vi "Hololens_GaitDisplay.vi"() -> ()   [LabVIEW 2016]
doc: "VI demonstrating how to add 3D objects to the Hololens space and to 3D Picture controls.\n\nHaro3D 2.2.0.7\nCopyright (c) 2018, HaroTek"
uses:
  Program Files (x86)/National Instruments/LabVIEW 2016/examples/HaroTek/Haro3D Examples/controls/_Hololens_3dobject_example_tab.ctl
  <vilib>/Utility/miscctls.llb/LV3DPointTypeDef.ctl
  <vilib>/HaroTek/Haro3D/Utilities/3D objects/controls/Material_info.ctl
  Program Files (x86)/National Instruments/LabVIEW 2016/examples/HaroTek/Haro3D Examples/Support/Holo_Example_Shape_ref_typedef.ctl
  <vilib>/HaroTek/Haro3D/Utilities/3D objects/3D_Shape_class/3D_Shape.lvclass
  C:/Program Files (x86)/National Instruments/LabVIEW 2016/vi.lib/HaroTek/Haro3D/Utilities/3D objects/3D_Object_class/3D_Object.lvclass
  <vilib>/HaroTek/Haro3D/Utilities/3D Operations/controls/_Deg_Rad_typedef.ctl
  <vilib>/HaroTek/Haro3D/Utilities/3D objects/Box_class/3D_Box.lvclass
  C:/Program Files (x86)/National Instruments/LabVIEW 2016/vi.lib/HaroTek/Haro3D/Utilities/3D objects/3D_Shape_class/3D_Shape.lvclass
  <vilib>/HaroTek/Haro3D/Utilities/3D objects/Cylinder_class/3D_Cylinder.lvclass
  <vilib>/HaroTek/Haro3D/Utilities/3D objects/Sphere_class/3D_Sphere_class/3D_Sphere.lvclass
  <vilib>/HaroTek/Haro3D/Utilities/3D objects/Mesh_class/Mesh.lvclass
  <vilib>/HaroTek/Haro3D/Utilities/3D objects/3D_Quad_class/Panel.lvclass
  <vilib>/picture/3D Picture Control/Object/Create Object (name).vi
  <vilib>/HaroTek/Haro3D/Utilities/3D objects/3D_Shape_class/properties/WriteMaterialInfo.vi
  <vilib>/HaroTek/Haro3D/Utilities/3D objects/3D_Object_class/properties/WritePosition.vi
  <vilib>/picture/3D Picture Control/Object/Add Object (reference).vi
  <vilib>/HaroTek/Haro3D/Utilities/3D objects/3D_Object_class/properties/ReadOrientation.vi
  <vilib>/HaroTek/Haro3D/Utilities/3D objects/OBJ classes/OBJ_Mesh_class/properties/ReadMeshArray.vi
  <vilib>/HaroTek/Haro3D/Utilities/3D objects/3D_Shape_class/properties/ReadShape.vi
  <vilib>/HaroTek/Haro3D/Utilities/3D objects/3D_Object_class/properties/ReadPosition.vi
  <vilib>/HaroTek/Haro3D/Utilities/3D objects/OBJ classes/OBJ_Mesh_class/OBJ_Mesh.lvclass
  <vilib>/HaroTek/Haro3D/Haro3D.lvlib
  <vilib>/picture/3D Picture Control/NI_3D Picture Control.lvlib
  <vilib>/HaroTek/Haro3D/Hololens/Hololens_class/Hololens.lvclass
  <vilib>/HaroTek/Haro3D/Hololens/Modules/Hololens Message classes/Object_Selected_Message_class/Object_Selected_Message.lvclass
  <vilib>/HaroTek/Haro3D/Hololens/Modules/Hololens Message classes/Mesh_Message_class/Mesh_Message.lvclass
panel:
  in  "Control container":enum32{"Page 2"}(tab)
  in  "Color":u32(colorbox)=16711680
  in  "Tab Control":T1
  in  "Cyl Length":sgl=0.3
  in  "Add Cylinder":bool
  in  "Cyl Radius":sgl=0.1
  in  "Cylinder info":string="Cylinder created in \nLabVIEW!"
  in  "Add Box":bool
  in  "Dimensions":T2={"X"=0.3, "Y"=0.2, "Z"=0.1}
  in  "Box Info":string="Box created in \nLabVIEW!"
  in  "Sphere Diameter":sgl=0.4
  in  "Add Sphere":bool
  in  "Sphere info":string="Sphere created in \nLabVIEW!"
  in  "Add Mesh":bool
  in  "Scale":dbl=1.0 format="%#_13g"
  in  "Panel":bool
  in  "Position":T2={"X"=0.0, "Y"=0.0, "Z"=2.0}
  in  "X rotation":sgl(slide) scale=-90.0..90.0
  in  "Y rotation":sgl(slide) scale=-180.0..270.0
  in  "Z rotation":sgl(slide) scale=-90.0..90.0
  in  "Pointer":bool
  in  "Reset View":bool
  out "Hololens":bool
  out "3D Picture":refnum<vi>(3d-picture)
  # "1. Start this VI and the Haro3D app on the Hololens\n2. Wait until the Hololens is connected to this VI.\n3. Use the tab to select a 3D object.\n4. Click to add the object to the Hololens and 3D Pict control\n5. Click again to modify the object properties\n6. Click the X to terminate the VI and the Hololens app."
  # "www.harotek.com"
  # "Scale is applied only when adding the mesh."
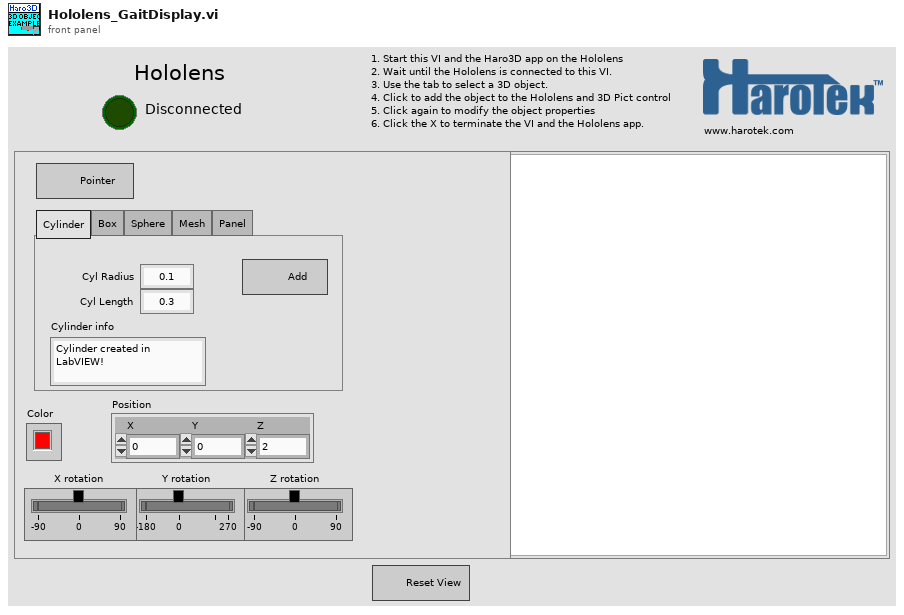
[diagram p1: front panel]
types:
  T1 = typedef "_Hololens_3dobject_example_tab.ctl" = enum32{"Cylinder", "Box", "Sphere", "Mesh", "Panel"}
  T2 = typedef "LV3DPointTypeDef.ctl" = cluster{"X":sgl, "Y":sgl, "Z":sgl}
  T3 = enum8{"Enabled", "Disabled", "Disabled and Grayed Out"}
  T4 = typedef "Holo_Example_Shape_ref_typedef.ctl" = cluster{"3D Pict":refnum<vi>, "hololens":refnum<class "3D_Shape.lvclass">}
  T5 = typedef "Haro3D.lvlib/Material_info.ctl" = cluster{"name":string, "Ka":u32, "Kd":u32, "Ke":u32, "Ks":u32, "map_Ka":string, "map_Kd":string, "map_Ks":string, "Ns":sgl, "Tr":sgl, "UseTexture":bool}
  T6 = cluster{"Connection":bool, "Position":T2, "Material info":T5, "Objects":T4[], "3D Picture":refnum<vi>, "Tab Control":T1}
  T7 = typedef "Haro3D.lvlib/Hololens.lvclass/Hololens_event.ctl" = cluster{"Connection":refnum<user-event>, "Data":refnum<user-event>}
  T8 = typedef "Haro3D.lvlib/_Deg_Rad_typedef.ctl" = enum16{"Deg", "Rad"}
  T9 = typedef "Haro3D.lvlib/Hololens.lvclass/data_event_type.ctl" = enum32{"None", "Mesh", "Text Response", "Manipulation", "Object selected", "Hold", "Receive Anchor", "Sharing", "Secondary connect", "Receive Picture", "Invalid"}
  T10 = typedef "quaternion.ctl" = cluster{"w":sgl, "x":sgl, "y":sgl, "z":sgl}
  T11 = typedef "Haro3D.lvlib/quaternion.ctl" = cluster{"w":sgl, "x":sgl, "y":sgl, "z":sgl}
  T12 = typedef "3D_Shape.lvclass/_shape_list_enum.ctl" = enum16{"None", "Cylinder", "Box", "Sphere", "Panel", "Mesh", "Texture_Mesh"}
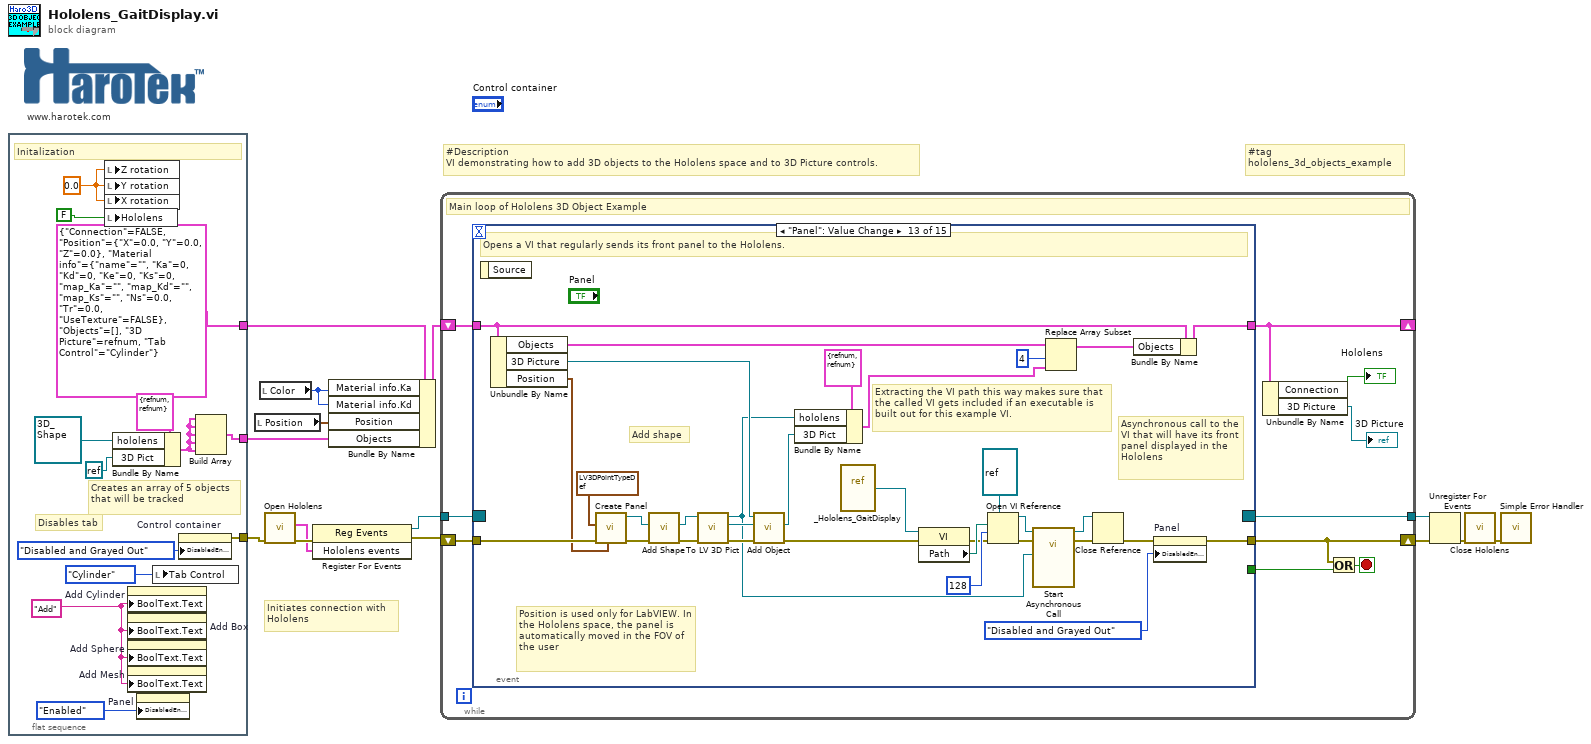
[diagram p0: block diagram]
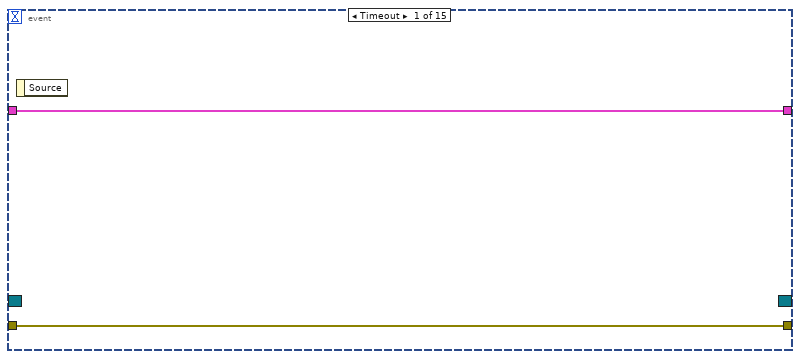
[diagram p2: hidden frame]
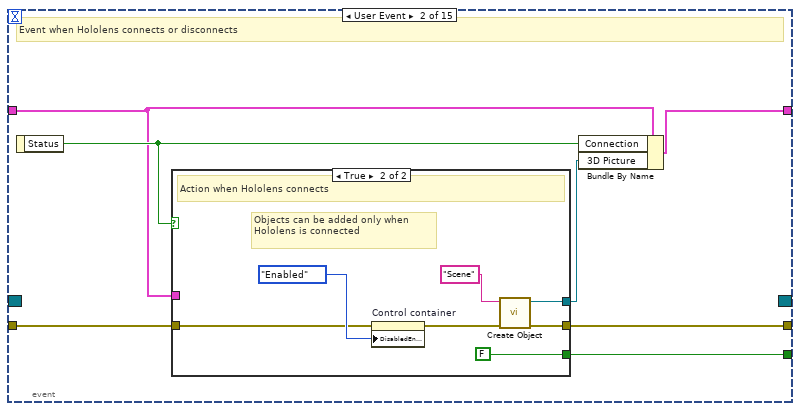
[diagram p3: hidden frame]
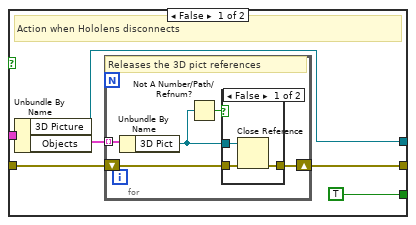
[diagram p4: hidden frame]
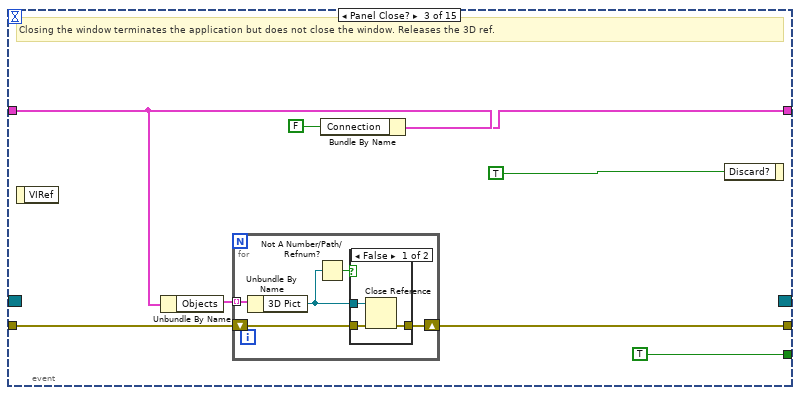
[diagram p6: hidden frame]
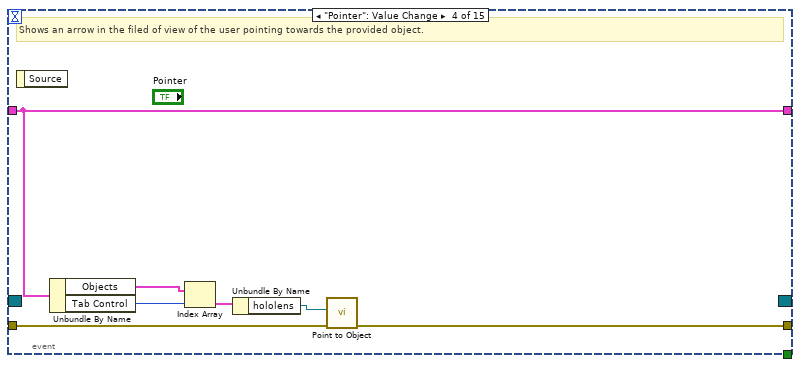
[diagram p8: hidden frame]
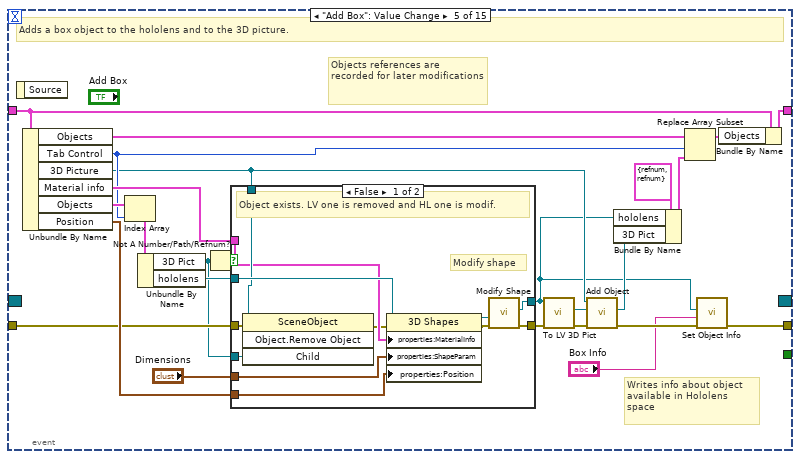
[diagram p9: hidden frame]
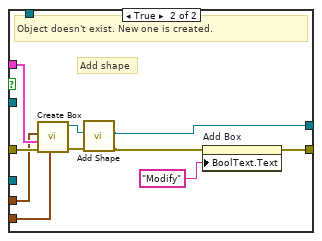
[diagram p10: hidden frame]
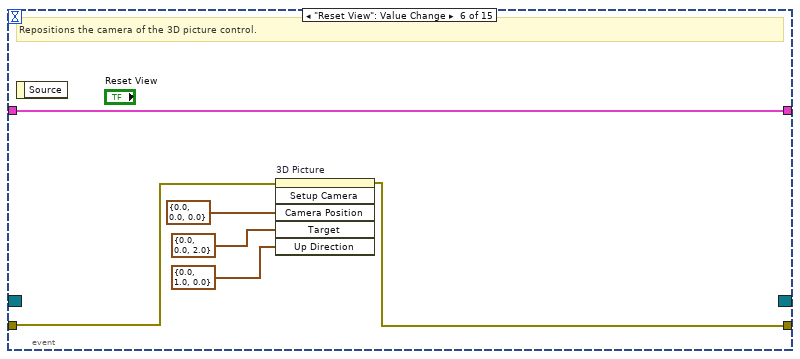
[diagram p11: hidden frame]
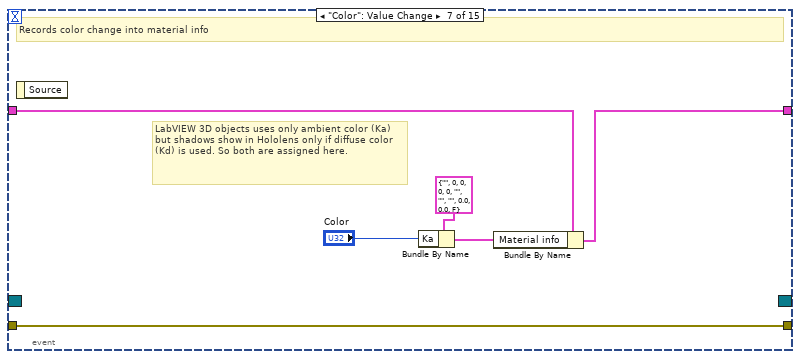
[diagram p12: hidden frame]
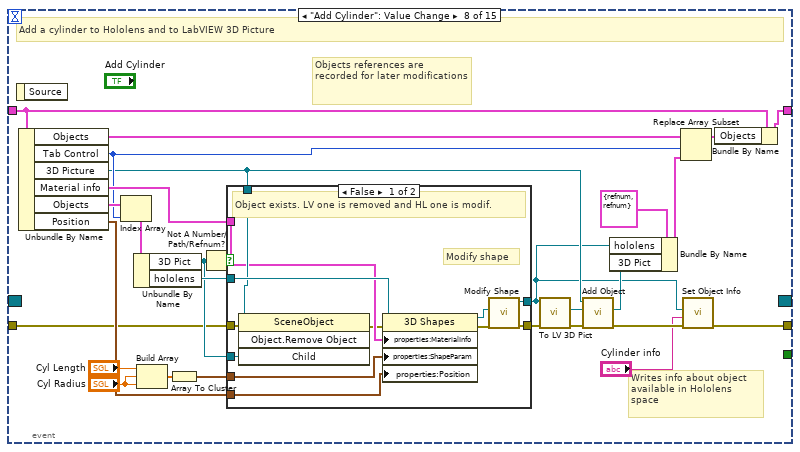
[diagram p13: hidden frame]
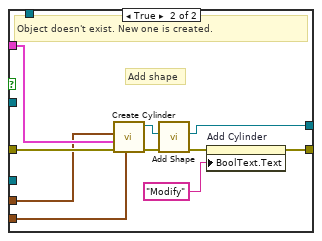
[diagram p14: hidden frame]
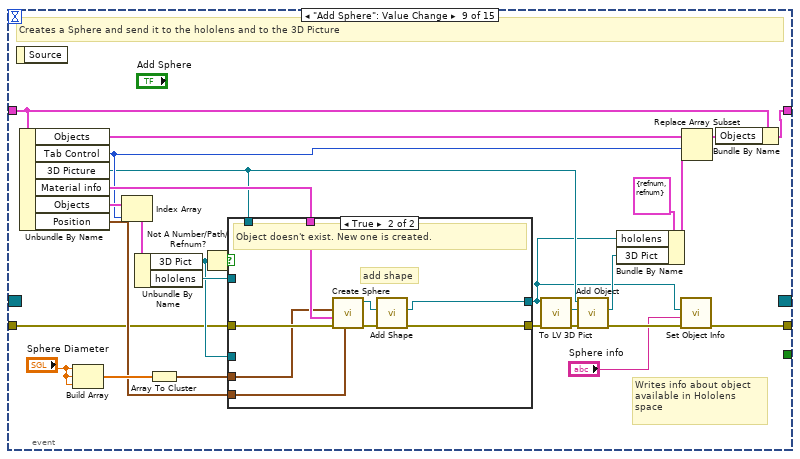
[diagram p15: hidden frame]
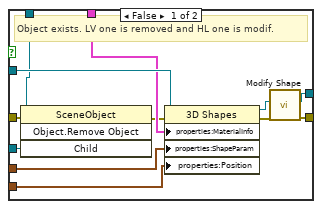
[diagram p16: hidden frame]
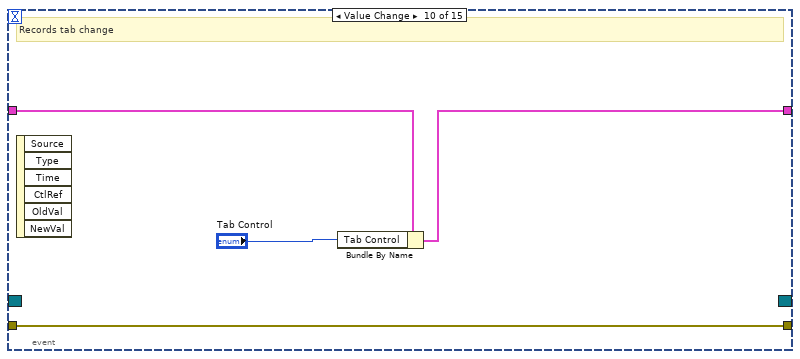
[diagram p17: hidden frame]
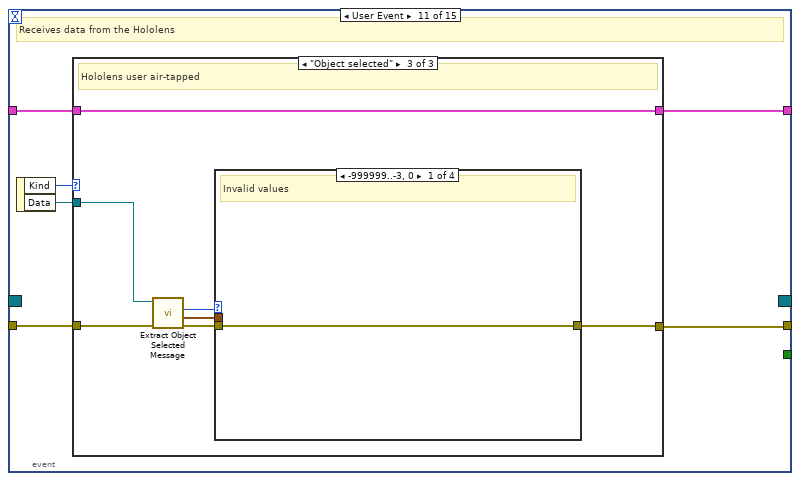
[diagram p18: hidden frame]
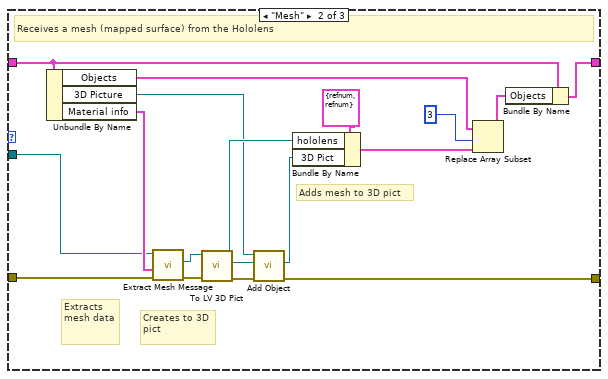
[diagram p20: hidden frame]
diagram:
  # "Initiates connection with\nHololens"
  # "www.harotek.com"
  # "#tag\nhololens_3d_objects_example"
  # "#Description\nVI demonstrating how to add 3D objects to the Hololens space and to 3D Picture controls."
  n1 = flat-sequence {
    tunnel: [w27] -> w7
    tunnel: [T6 {"Connection"=FALSE, "Position"={"X"=0.0, "Y"=0.0, "Z"=0.0}, "Material info"={"name"="", "Ka"=0, "Kd"=0, "Ke"=0, "Ks"=0, "map_Ka"="", "map_Kd"="", "map_Ks"="", "Ns"=0.0, "Tr"=0.0, "UseTexture"=FALSE}, "Objects"=[], "3D Picture"=refnum, "Tab Control"=enum."Cylinder"}] -> w10
    tunnel: [w24] -> w9
    frame #0 {
      w19 = "Add" ("Boolean Text.Text")
      w20 = sgl 0.0 ("Z rotation")
      # "Disables tab"
      # "Creates an array of 5 objects that will be tracked"
      # "Initalization"
      n2 = local write "Z rotation"(w20) -> ()
      n3 = local write "Y rotation"(w20) -> ()
      n4 = local write "X rotation"(w20) -> ()
      n5 = local write "Hololens"(FALSE) -> ()
      n6 = Bundle By Name(cluster=T4 {"3D Pict"=refnum, "hololens"=refnum}, "hololens"=refnum<class "3D_Shape.lvclass"> refnum ("3D Shapes"), "3D Pict"=refnum<k0> refnum) -> (w16:T4)
      n7 = property on="Add Cylinder" class="Bool"("BoolText.Text"=w19) -> ()  [unwired: 2 in, 2 out]
      n8 = property on="Add Box" class="Bool"("BoolText.Text"=w19) -> ()  [unwired: 2 in, 2 out]
      n9 = property on="Add Sphere" class="Bool"("BoolText.Text"=w19) -> ()  [unwired: 2 in, 2 out]
      n10 = property on="Add Mesh" class="Bool"("BoolText.Text"=w19) -> ()  [unwired: 2 in, 2 out]
      n11 = property on="Panel" class="Bool"("DisabledEnum"=T3."Enabled" ("Disabled")) -> ()  [unwired: 2 in, 2 out]
      n12 = local write "Tab Control"(_Hololens_3dobject_example_tab."Cylinder" ("Tab Control")) -> ()
      n13 = property on="Control container" class="TabCtl (strict)"("DisabledEnum"=T3."Disabled and Grayed Out" ("Disabled")) -> (error out=w27:errorcluster)  [unwired: 2 in, 1 out]
      n14 = Build Array(w16, w16, w16, w16, w16) -> (w24:T4[])
    }
  }
  n15 = local read "Position"() -> (w11:T2)
  n16 = local read "Color"() -> (w8:u32)
  n17 = call <vilib>:"Open Hololens.vi"("error in (no error)"=w7) -> ("error out"=w6:errorcluster, "Hololens events"=w5:T7)  [unwired: 9 in]
  n18 = register-events(error in=w6, w5) -> (reference out=w3:refnum<event-registration>, error out=w4:errorcluster)  [unwired: 1 in]
  n19 = Bundle By Name(cluster=w10, "Material info.Ka"=w8, "Material info.Kd"=w8, "Position"=w11, "Objects"=w9) -> (w12:T6)
  n20 = while {
    shift-right: [w34] -> _
    shift-left: w12 -> [w37]
    tunnel: [w36] -> w14
    shift-right: [w29] -> w13
    shift-left: w4 -> [w35]
    tunnel: w3 -> [w28]
    stop <- w30 stop-if-true
    # "Main loop of Hololens 3D Object Example"
    n21 = event shown="[12] \"Panel\": Value Change" {
      selector: w28 -> [_ _ _ _ _ _ _ _ _ _ _ _ _ _ _]
      dyn-events: [_ _ _ _ _ _ _ _ _ _ _ _ _ _ _] -> w36
      timeout: _ -> [_ _ _ _ _ _ _ _ _ _ _ _ _ _ _]
      tunnel: w37 -> [w38 w41 w72 w86 w115 w140 w151 w159 w208 w252 w255 w321 w383 w396 w442]
      tunnel: w35 -> [w39 w45 w75 w92 w106 w141 w149 w156 w206 w249 w256 w320 w373 w404 w439]
      tunnel: [w39 w42 w76 w91 w94 w142 w149 w154 w204 w249 w253 w318 w387 w392 w439] -> w29
      tunnel: [w38 w46 w71 w86 w114 w140 w150 w158 w209 w251 w254 w316 w363 w395 w441] -> w34
      tunnel: [_ w43 TRUE _ _ _ _ _ _ _ _ _ _ _ _] -> w31
      event Timeout {
        n22 = event-data() -> ()  [unwired: 1 in, 1 out]
      }
      event User Event {
        # "Event when Hololens connects or disconnects"
        n23 = event-data() -> ("Status"=w44:bool)  [unwired: 1 in]
        n24 = case shown="True" w44 {
          tunnel: w45 -> [w49 w66]
          tunnel: [TRUE FALSE] -> w43
          tunnel: [w50 w64] -> w42
          tunnel: w41 -> [w48 _]
          tunnel: [w47 w63] -> w40
          frame False {
            # "Action when Hololens disconnects"
            n25 = Unbundle By Name(w48) -> ("3D Picture"=w47:refnum<vi>, "Objects"=w51:T4[])
            n26 = for {
              shift-right: [w57] -> w50
              shift-left: w49 -> [w56]
              tunnel: w51 -> [w55] mode=indexing
              # "Releases the 3D pict references"
              n27 = Unbundle By Name(w55) -> ("3D Pict"=w54:refnum<vi>)
              n28 = Not A Number/Path/Refnum?(number/path/refnum=w54) -> (NaN/Path/Refnum?=w53:bool)
              n29 = case shown="False" w53 {
                tunnel: [w60 w61] -> w57
                tunnel: w56 -> [w59 w61]
                tunnel: w54 -> [w58 _]
                frame False {
                  n30 = Close Reference(reference=w58, error in (no error)=w59) -> (error out=w60:errorcluster)
                }
                frame True {
                }
              }
            }
          }
          frame True {
            # "Objects can be added only when Hololens is connected"
            # "Action when Hololens connects"
            n31 = property on="Control container" class="TabCtl (strict)"(error in=w66, "DisabledEnum"=T3."Enabled" ("Disabled")) -> (error out=w65:errorcluster)  [unwired: 1 in, 1 out]
            n32 = call-poly <vilib>:"Create Object.vi"("error in (no error)"=w65, "Name"="Scene") -> ("error out"=w64:errorcluster, "Scene:New Object"=w63:refnum<vi>)  [unwired: 8 in]
          }
        }
        n33 = Bundle By Name(cluster=w41, "Connection"=w44, "3D Picture"=w40) -> (w46:T6)
      }
      event Panel Close? {
        # "Closing the window terminates the application but does not close the window. Releases the 3D ref."
        n34 = event-data() -> ()  [unwired: 1 in, 1 out]
        n35 = Unbundle By Name(w72) -> ("Objects"=w74:T4[])
        n36 = for {
          shift-right: [w81] -> w76
          shift-left: w75 -> [w80]
          tunnel: w74 -> [w79] mode=indexing
          n37 = Unbundle By Name(w79) -> ("3D Pict"=w78:refnum<vi>)
          n38 = Not A Number/Path/Refnum?(number/path/refnum=w78) -> (NaN/Path/Refnum?=w77:bool)
          n39 = case shown="False" w77 {
            tunnel: [w84 w85] -> w81
            tunnel: w80 -> [w83 w85]
            tunnel: w78 -> [w82 _]
            frame False {
              n40 = Close Reference(reference=w82, error in (no error)=w83) -> (error out=w84:errorcluster)
            }
            frame True {
            }
          }
        }
        n41 = Bundle By Name(cluster=w72, "Connection"=FALSE) -> (w71:T6)
        n42 = event-data("Discard?"=TRUE) -> ()  [unwired: 1 in, 1 out]
      }
      event "Pointer": Value Change {
        # "Shows an arrow in the filed of view of the user pointing towards the provided object."
        n43 = event-data() -> ()  [unwired: 1 in, 1 out]
        n44 = Unbundle By Name(w86) -> ("Objects"=w89:T4[], "Tab Control"=w90:T1)
        n45 = Index Array(array=w89, index=w90) -> (element=w88:T4)
        n46 = Unbundle By Name(w88) -> ("hololens"=w87:refnum<class "3D_Shape.lvclass">)
        n47 = call <vilib>:"Point to Object.vi"("error in (no error)"=w92, "3D Object (hides)"=w87) -> ("error out"=w91:errorcluster)  [unwired: 9 in]
      }
      event "Add Box": Value Change {
        # "Writes info about object available in Hololens space"
        # "Objects references are recorded for later modifications"
        # "Adds a box object to the hololens and to the 3D picture."
        n48 = event-data() -> ()  [unwired: 1 in, 1 out]
        n49 = Unbundle By Name(w115) -> ("Objects"=w112:T4[], "Tab Control"=w108:T1, "3D Picture"=w99:refnum<vi>, "Material info"=w117:T5, "Objects"=w109:T4[], "Position"=w116:T2)
        n50 = Index Array(array=w109, index=w108) -> (element=w107:T4)
        n51 = Unbundle By Name(w107) -> ("3D Pict"=w100:refnum<vi>, "hololens"=w103:refnum<class "3D_Shape.lvclass">)
        n52 = Not A Number/Path/Refnum?(number/path/refnum=w100) -> (NaN/Path/Refnum?=w104:bool)
        n53 = case shown="False" w104 {
          tunnel: w117 -> [w125 w139]
          tunnel: w116 -> [w122 w138]
          tunnel: [w121 w134] -> w101
          tunnel: w106 -> [w129 w137]
          tunnel: "Dimensions" -> [w124 w136]
          tunnel: w103 -> [w128 _]
          tunnel: [w118 w132] -> w96
          tunnel: w100 -> [w127 _]
          tunnel: w99 -> [w126 _]
          frame False {
            # "Modify shape"
            # "Object exists. LV one is removed and HL one is modif."
            n54 = invoke class="SceneObject" method="Object.Remove Object"(reference=w126, error in=w129, "Child"=w127) -> (error out=w123:errorcluster)  [unwired: 1 in, 3 out]
            n55 = property class="3D Shapes"(reference=w128, error in=w123, "properties:MaterialInfo"=w125, "properties:ShapeParam"=w124, "properties:Position"=w122) -> (reference out=w119:refnum<class "3D_Shape.lvclass">, error out=w120:errorcluster)
            n56 = call <vilib>:"Modify Shape.vi"("error in (no error)"=w120, "Shape in"=w119) -> ("error out"=w121:errorcluster, "Shape out"=w118:refnum<class "3D_Shape.lvclass">)  [unwired: 8 in]
          }
          frame True {
            # "Add shape"
            # "Object doesn't exist. New one is created."
            n57 = call <vilib>:"Create Box.vi"("Position"=w138, "error in (no error)"=w137, "Material info"=w139, "Dimensions"=w136) -> ("error out"=w133:errorcluster, "Box out"=w130:refnum<class "3D_Box.lvclass">)  [unwired: 6 in]
            n58 = call <vilib>:"Add Shape.vi"("error in (no error)"=w133, "Shape in"=w130) -> ("error out"=w131:errorcluster, "Shape out"=w132:refnum<class "3D_Box.lvclass">)  [unwired: 7 in, 1 out]
            n59 = property on="Add Box" class="Bool"(error in=w131, "BoolText.Text"="Modify" ("Boolean Text.Text")) -> (error out=w134:errorcluster)  [unwired: 1 in, 1 out]
          }
        }
        n60 = call-dynamic "To LV 3D Pict.vi"("error in (no error)"=w101, "3D object in"=w96) -> ("error out"=w102:errorcluster, "LabVIEW 3D Object ref"=w97:refnum<vi>)  [unwired: 7 in, 1 out]
        n61 = call-poly <vilib>:"Add Object.vi"("error in (no error)"=w102, "New Object In"=w97, "Scene Object In"=w99) -> ("error out"=w95:errorcluster, "New Object Out"=w98:refnum<vi>)  [unwired: 6 in, 1 out]
        n62 = Bundle By Name(cluster=T4 {"3D Pict"=refnum, "hololens"=refnum}, "hololens"=w96, "3D Pict"=w98) -> (w111:T4)
        n63 = Replace Array Subset(array=w112, new element=w111, index=w108) -> (w113:T4[])
        n64 = call <vilib>:"Set Object Info.vi"("error in (no error)"=w95, "Text"="Box Info", "Shape"=w96) -> ("error out"=w94:errorcluster)  [unwired: 8 in]
        n65 = Bundle By Name(cluster=w115, "Objects"=w113) -> (w114:T6)
      }
      event "Reset View": Value Change {
        # "Repositions the camera of the 3D picture control."
        n66 = event-data() -> ()  [unwired: 1 in, 1 out]
        n67 = invoke on="3D Picture" class="SceneGraphDisp (strict)" method="Setup Camera"(error in=w141, "Camera Position"=T2 {"X"=0.0, "Y"=0.0, "Z"=0.0}, "Target"=T2 {"X"=0.0, "Y"=0.0, "Z"=2.0}, "Up Direction"=T2 {"X"=0.0, "Y"=1.0, "Z"=0.0}) -> (error out=w142:errorcluster)  [unwired: 2 in, 5 out]
      }
      event "Color": Value Change {
        # "LabVIEW 3D objects uses only ambient color (Ka) but shadows show in Hololens only if diffuse color (Kd) is used. So both are assigned here."
        # "Records color change into material info"
        n68 = event-data() -> ()  [unwired: 1 in, 1 out]
        n69 = Bundle By Name(cluster=T5 {"name"="", "Ka"=0, "Kd"=0, "Ke"=0, "Ks"=0, "map_Ka"="", "map_Kd"="", "map_Ks"="", "Ns"=0.0, "Tr"=0.0, "UseTexture"=FALSE} ("Material info"), "Ka"="Color") -> (w148:T5)
        n70 = Bundle By Name(cluster=w151, "Material info"=w148) -> (w150:T6)
      }
      event "Add Cylinder": Value Change {
        # "Writes info about object available in Hololens space"
        # "Objects references are recorded for later modifications"
        # "Add a cylinder to Hololens and to LabVIEW 3D Picture"
        n71 = event-data() -> ()  [unwired: 1 in, 1 out]
        n72 = Unbundle By Name(w159) -> ("Objects"=w173:T4[], "Tab Control"=w169:T1, "3D Picture"=w162:refnum<vi>, "Material info"=w176:T5, "Objects"=w170:T4[], "Position"=w175:T2)
        n73 = Index Array(array=w170, index=w169) -> (element=w168:T4)
        n74 = Unbundle By Name(w168) -> ("3D Pict"=w163:refnum<vi>, "hololens"=w166:refnum<class "3D_Shape.lvclass">)
        n75 = Build Array("Cyl Length", "Cyl Radius", "Cyl Radius") -> (w177:sgl[])
        n76 = Array To Cluster(array=w177) -> (cluster=w155:cluster{"[0]":sgl, "[1]":sgl, "[2]":sgl})
        n77 = Not A Number/Path/Refnum?(number/path/refnum=w163) -> (NaN/Path/Refnum?=w167:bool)
        n78 = case shown="False" w167 {
          tunnel: w176 -> [w187 w201]
          tunnel: w175 -> [w184 w200]
          tunnel: [w182 w196] -> w164
          tunnel: w156 -> [w191 w199]
          tunnel: w155 -> [w186 w198]
          tunnel: w166 -> [w190 _]
          tunnel: [w181 w192] -> w153
          tunnel: w163 -> [w189 _]
          tunnel: w162 -> [w188 _]
          frame False {
            # "Modify shape"
            # "Object exists. LV one is removed and HL one is modif."
            n79 = invoke class="SceneObject" method="Object.Remove Object"(reference=w188, error in=w191, "Child"=w189) -> (error out=w185:errorcluster)  [unwired: 1 in, 3 out]
            n80 = property class="3D Shapes"(reference=w190, error in=w185, "properties:MaterialInfo"=w187, "properties:ShapeParam"=w186, "properties:Position"=w184) -> (reference out=w180:refnum<class "3D_Shape.lvclass">, error out=w183:errorcluster)
            n81 = call <vilib>:"Modify Shape.vi"("error in (no error)"=w183, "Shape in"=w180) -> ("error out"=w182:errorcluster, "Shape out"=w181:refnum<class "3D_Shape.lvclass">)  [unwired: 8 in]
          }
          frame True {
            # "Add shape"
            # "Object doesn't exist. New one is created."
            n82 = call <vilib>:"Create Cylinder.vi"("Position"=w200, "error in (no error)"=w199, "Material info"=w201, "Dimensions"=w198) -> ("error out"=w195:errorcluster, "Cylinder out"=w194:refnum<class "3D_Cylinder.lvclass">)  [unwired: 6 in]
            n83 = call <vilib>:"Add Shape.vi"("error in (no error)"=w195, "Shape in"=w194) -> ("error out"=w193:errorcluster, "Shape out"=w192:refnum<class "3D_Cylinder.lvclass">)  [unwired: 7 in, 1 out]
            n84 = property on="Add Cylinder" class="Bool"(error in=w193, "BoolText.Text"="Modify" ("Boolean Text.Text")) -> (error out=w196:errorcluster)  [unwired: 1 in, 1 out]
          }
        }
        n85 = call-dynamic "To LV 3D Pict.vi"("error in (no error)"=w164, "3D object in"=w153) -> ("error out"=w165:errorcluster, "LabVIEW 3D Object ref"=w160:refnum<vi>)  [unwired: 7 in, 1 out]
        n86 = call-poly <vilib>:"Add Object.vi"("error in (no error)"=w165, "New Object In"=w160, "Scene Object In"=w162) -> ("error out"=w157:errorcluster, "New Object Out"=w161:refnum<vi>)  [unwired: 6 in, 1 out]
        n87 = Bundle By Name(cluster=T4 {"3D Pict"=refnum, "hololens"=refnum}, "hololens"=w153, "3D Pict"=w161) -> (w172:T4)
        n88 = Replace Array Subset(array=w173, new element=w172, index=w169) -> (w174:T4[])
        n89 = call <vilib>:"Set Object Info.vi"("error in (no error)"=w157, "Text"="Cylinder info", "Shape"=w153) -> ("error out"=w154:errorcluster)  [unwired: 8 in]
        n90 = Bundle By Name(cluster=w159, "Objects"=w174) -> (w158:T6)
      }
      event "Add Sphere": Value Change {
        # "Writes info about object available in Hololens space"
        # "Creates a Sphere and send it to the hololens and to the 3D Picture"
        n91 = event-data() -> ()  [unwired: 1 in, 1 out]
        n92 = Unbundle By Name(w208) -> ("Objects"=w223:T4[], "Tab Control"=w219:T1, "3D Picture"=w212:refnum<vi>, "Material info"=w226:T5, "Objects"=w220:T4[], "Position"=w225:T2)
        n93 = Build Array("Sphere Diameter", "Sphere Diameter", "Sphere Diameter") -> (w227:sgl[])
        n94 = Index Array(array=w220, index=w219) -> (element=w218:T4)
        n95 = Unbundle By Name(w218) -> ("3D Pict"=w213:refnum<vi>, "hololens"=w216:refnum<class "3D_Shape.lvclass">)
        n96 = Array To Cluster(array=w227) -> (cluster=w205:cluster{"[0]":sgl, "[1]":sgl, "[2]":sgl})
        n97 = Not A Number/Path/Refnum?(number/path/refnum=w213) -> (NaN/Path/Refnum?=w217:bool)
        n98 = case shown="True" w217 {
          tunnel: w226 -> [w236 w248]
          tunnel: w225 -> [w233 w247]
          tunnel: [w230 w243] -> w214
          tunnel: w206 -> [w240 w246]
          tunnel: w205 -> [w235 w245]
          tunnel: w216 -> [w239 _]
          tunnel: [w229 w242] -> w202
          tunnel: w213 -> [w238 _]
          tunnel: w212 -> [w237 _]
          frame False {
            # "Object exists. LV one is removed and HL one is modif."
            n99 = invoke class="SceneObject" method="Object.Remove Object"(reference=w237, error in=w240, "Child"=w238) -> (error out=w234:errorcluster)  [unwired: 1 in, 3 out]
            n100 = property class="3D Shapes"(reference=w239, error in=w234, "properties:MaterialInfo"=w236, "properties:ShapeParam"=w235, "properties:Position"=w233) -> (reference out=w231:refnum<class "3D_Shape.lvclass">, error out=w232:errorcluster)
            n101 = call <vilib>:"Modify Shape.vi"("error in (no error)"=w232, "Shape in"=w231) -> ("error out"=w230:errorcluster, "Shape out"=w229:refnum<class "3D_Shape.lvclass">)  [unwired: 8 in]
          }
          frame True {
            # "add shape"
            # "Object doesn't exist. New one is created."
            n102 = call <vilib>:"Create Sphere.vi"("Position"=w247, "error in (no error)"=w246, "Material info"=w248, "Dimensions"=w245) -> ("error out"=w244:errorcluster, "Sphere out"=w241:refnum<class "3D_Sphere.lvclass">)  [unwired: 6 in]
            n103 = call <vilib>:"Add Shape.vi"("error in (no error)"=w244, "Shape in"=w241) -> ("error out"=w243:errorcluster, "Shape out"=w242:refnum<class "3D_Sphere.lvclass">)  [unwired: 7 in, 1 out]
          }
        }
        n104 = call-dynamic "To LV 3D Pict.vi"("error in (no error)"=w214, "3D object in"=w202) -> ("error out"=w215:errorcluster, "LabVIEW 3D Object ref"=w210:refnum<vi>)  [unwired: 7 in, 1 out]
        n105 = call-poly <vilib>:"Add Object.vi"("error in (no error)"=w215, "New Object In"=w210, "Scene Object In"=w212) -> ("error out"=w207:errorcluster, "New Object Out"=w211:refnum<vi>)  [unwired: 6 in, 1 out]
        n106 = Bundle By Name(cluster=T4 {"3D Pict"=refnum, "hololens"=refnum}, "hololens"=w202, "3D Pict"=w211) -> (w222:T4)
        n107 = call <vilib>:"Set Object Info.vi"("error in (no error)"=w207, "Text"="Sphere info", "Shape"=w202) -> ("error out"=w204:errorcluster)  [unwired: 8 in]
        n108 = Replace Array Subset(array=w223, new element=w222, index=w219) -> (w224:T4[])
        n109 = Bundle By Name(cluster=w208, "Objects"=w224) -> (w209:T6)
      }
      event Value Change {
        # "Records tab change"
        n110 = event-data() -> ()  [unwired: 1 in, 6 out]
        n111 = Bundle By Name(cluster=w252, "Tab Control"="Tab Control") -> (w251:T6)
      }
      event User Event {
        # "Receives data from the Hololens"
        n112 = event-data() -> ("Kind"=w258:T9, "Data"=w257:refnum<class "Holo_Event_Data.lvclass">)  [unwired: 1 in]
        n113 = case shown="\"Object selected\"" w258 {
          tunnel: w257 -> [_ w262 w281]
          tunnel: w256 -> [w259 w264 w283]
          tunnel: w255 -> [w260 w272 w284]
          tunnel: [w260 w270 w284] -> w254
          tunnel: [w259 w266 w285] -> w253
          frame "None", Default {
          }
          frame "Mesh" {
            # "Adds mesh to 3D pict"
            # "Creates to 3D pict"
            # "Extracts mesh data"
            # "Receives a mesh (mapped surface) from the Hololens"
            n114 = Unbundle By Name(w272) -> ("Objects"=w273:T4[], "3D Picture"=w274:refnum<vi>, "Material info"=w263:T5)
            n115 = call <vilib>:"Extract Mesh Message.vi"("error in (no error)"=w264, "Material info"=w263, "Generic Event Message"=w262) -> ("error out"=w265:errorcluster, "Mesh object"=w261:refnum<class "Mesh.lvclass">)  [unwired: 4 in, 3 out]
            n116 = call-dynamic "To LV 3D Pict.vi"("error in (no error)"=w265, "Mesh in"=w261) -> ("error out"=w269:errorcluster, "LabVIEW 3D object ref"=w268:refnum<vi>, "Mesh out"=w278:refnum<class "Mesh.lvclass">)  [unwired: 7 in]
            n117 = call-poly <vilib>:"Add Object.vi"("error in (no error)"=w269, "New Object In"=w268, "Scene Object In"=w274) -> ("error out"=w266:errorcluster, "New Object Out"=w277:refnum<vi>)  [unwired: 6 in, 1 out]
            n118 = Bundle By Name(cluster=T4 {"3D Pict"=refnum, "hololens"=refnum}, "hololens"=w278, "3D Pict"=w277) -> (w276:T4)
            n119 = Replace Array Subset(array=w273, new element=w276, index=3) -> (w271:T4[])
            n120 = Bundle By Name(cluster=w272, "Objects"=w271) -> (w270:T6)
          }
          frame "Object selected" {
            # "Hololens user air-tapped"
            n121 = call <vilib>:"Extract Object Selected Message.vi"("error in (no error)"=w283, "Generic message"=w281) -> ("error out"=w282:errorcluster, "Cursor position"=w280:cluster{"X":sgl, "Y":sgl, "Z":sgl}, "Object"=w279:i32)  [unwired: 5 in, 2 out]
            n122 = case shown="-999999..-3, 0" w279 {
              selector: w279 -> [_ _ w293 _]
              tunnel: w282 -> [w286 w287 w297 w299]
              tunnel: w280 -> [_ _ _ w298]
              tunnel: [w286 w287 w290 w300] -> w285
              frame -999999..-3, 0 {
                # "Invalid values"
              }
              frame -2 {
                # "Object other than mapped surface or LabVIEW. No action"
              }
              frame 1, Default {
                # "Mod\nMulti materials"
                # "Generic 3D shape"
                # "LabVIEW object. Changes color to purple."
                n123 = Bundle By Name(cluster=T5 {"name"="", "Ka"=0, "Kd"=0, "Ke"=0, "Ks"=0, "map_Ka"="", "map_Kd"="", "map_Ks"="", "Ns"=0.0, "Tr"=0.0, "UseTexture"=FALSE} ("MaterialInfo"), "Kd"=u32 12976383) -> (w294:T5)
                n124 = property class="3D Shapes"(reference=refnum<class "3D_Shape.lvclass"> refnum ("3D Shapes"), error in=w297, "properties:HoloIndex"=w293, "properties:MaterialInfo"=w294) -> (reference out=w292:refnum<class "3D_Shape.lvclass">, error out=w289:errorcluster)
                n125 = Build Array(w292) -> (w288:refnum<class "3D_Shape.lvclass">[])
                n126 = call <vilib>:"Modify Multi Materials.vi"("error in (no error)"=w289, "Shape array"=w288) -> ("error out"=w290:errorcluster)  [unwired: 9 in]
              }
              frame -1 {
                # "Move origin"
                # "Air-tapped object is a mapped surface. Moves origin at that point"
                n127 = call <vilib>:"Move Origin.vi"("error in (no error)"=w299, "Position"=w298) -> ("error out"=w300:errorcluster)  [unwired: 9 in]
              }
            }
          }
        }
      }
      event "Add Mesh": Value Change {
        # "Checks if the mesh already exists"
        # "Once created, Hololens object cannot be deleted. They can only be hidden or modified."
        # "Loads a mesh from a .obj file and displays it in the Hololens and in the LabVIEW 3D Picture."
        n128 = event-data() -> ()  [unwired: 1 in, 1 out]
        n129 = Unbundle By Name(w321) -> ("Material info"=w303:T5, "Objects"=w308:T4[], "3D Picture"=w302:refnum<vi>, "Position"=w317:T2)
        n130 = Index Array(array=w308, index=3) -> (element=w309:T4)
        n131 = Unbundle By Name(w309) -> ("3D Pict"=w304:refnum<vi>, "hololens"=w306:refnum<class "3D_Shape.lvclass">)
        n132 = Not A Number/Path/Refnum?(number/path/refnum=w304) -> (NaN/Path/Refnum?=w305:bool)
        n133 = case shown="True" w305 {
          tunnel: w320 -> [w335 w352]
          tunnel: [w331 w351] -> w319
          tunnel: w317 -> [w325 w347]
          tunnel: [w330 w344] -> w301
          tunnel: [w329 w343] -> w313
          tunnel: w306 -> [w333 _]
          tunnel: w304 -> [w332 _]
          tunnel: w303 -> [w326 _]
          tunnel: w302 -> [w328 _]
          frame False {
            n134 = invoke class="SceneObject" method="Object.Remove Object"(reference=w328, error in=w335, "Child"=w332) -> (error out=w337:errorcluster)  [unwired: 1 in, 3 out]
            n135 = property class="3D Shapes"(reference=w333, error in=w337, "properties:MaterialInfo"=w326) -> (reference out=w323:refnum<class "3D_Shape.lvclass">, error out=w336:errorcluster, "properties:Orientation"=w324:T10)
            n136 = call <vilib>:"Move Object.vi"("Quaternion (no rotation)"=w324, "Position"=w325, "3D Object in"=w323) -> ("3D Object out"=w322:refnum<class "3D_Shape.lvclass">)  [unwired: 7 in, 1 out]
            n137 = Build Array(w322) -> (w327:refnum<class "3D_Shape.lvclass">[])
            n138 = call <vilib>:"Modify Multi Materials.vi"("error in (no error)"=w336, "Shape array"=w327) -> ("error out"=w334:errorcluster)  [unwired: 9 in]
            n139 = call-dynamic "To LV 3D Pict.vi"("error in (no error)"=w334, "3D object in"=w322) -> ("error out"=w331:errorcluster, "LabVIEW 3D Object ref"=w329:refnum<vi>, "3D Object out"=w330:refnum<class "3D_Shape.lvclass">)  [unwired: 7 in]
          }
          frame True {
            # "Send OBJ Mesh to Hololens"
            n140 = Current VI's Path() -> (path=w355:path)
            n141 = Strip Path(path=w355) -> (stripped path=w350:path)  [unwired: 1 out]
            n142 = Build Path(base path=w350, name or relative path=path "Support/astronaut/astronaut.obj") -> (appended path=w353:path)
            n143 = call <vilib>:"OBJ_File_Load.vi"("Position (0,0,0)"=w347, "Scale (1)"="Scale", "error in (no error)"=w352, "Path"=w353) -> ("error out"=w341:errorcluster, "OBJ object"=w340:refnum<class "OBJ_Mesh.lvclass">)  [unwired: 6 in]
            n144 = call-dynamic "Send to Hololens.vi"("error in (no error)"=w341, "OBJ object in"=w340) -> ("error out"=w338:errorcluster, "OBJ object out"=w339:refnum<class "OBJ_Mesh.lvclass">)  [unwired: 8 in]
            n145 = property class="OBJ_Mesh"(reference=w339) -> ("properties:MeshArray"=w345:refnum<class "Mesh.lvclass">[])  [unwired: 1 in, 2 out]
            n146 = call <vilib>:"Calculate Normals.vi"("error in (no error)"=w338, "OBJ_Mesh in"=w339) -> ("error out"=w349:errorcluster, "OBJ_Mesh out"=w348:refnum<class "OBJ_Mesh.lvclass">)  [unwired: 8 in]
            n147 = property on="Add Mesh" class="Bool"("BoolText.Text"="Modify" ("Boolean Text.Text")) -> ()  [unwired: 2 in, 2 out]
            n148 = call-dynamic "To LV 3D Pict.vi"("error in (no error)"=w349, "OBJ Mesh in"=w348) -> ("error out"=w351:errorcluster, "LabVIEW 3D object ref"=w343:refnum<vi>)  [unwired: 7 in, 1 out]
            n149 = Index Array(array=w345) -> (element=w344:refnum<class "Mesh.lvclass">)  [unwired: 1 in]
          }
        }
        n150 = call-poly <vilib>:"Add Object.vi"("error in (no error)"=w319, "New Object In"=w313, "Scene Object In"=w302) -> ("error out"=w318:errorcluster, "New Object Out"=w310:refnum<vi>)  [unwired: 6 in, 1 out]
        n151 = Bundle By Name(cluster=T4 {"3D Pict"=refnum, "hololens"=refnum} ("new element/subarray"), "hololens"=w301, "3D Pict"=w310) -> (w312:T4)
        n152 = Replace Array Subset(array=w308, new element=w312, index=3) -> (w315:T4[])
        n153 = Bundle By Name(cluster=w321, "Objects"=w315) -> (w316:T6)
      }
      event "Panel": Value Change {
        # "Add shape"
        # "Extracting the VI path this way makes sure that the called VI gets included if an executable is built out for this example VI."
        # "Asynchronous call to the VI that will have its front panel displayed in the Hololens"
        # "Position is used only for LabVIEW. In the Hololens space, the panel is automatically moved in the FOV of the user"
        # "Opens a VI that regularly sends its front panel to the Hololens."
        n154 = event-data() -> ()  [unwired: 1 in, 1 out]
        n155 = Unbundle By Name(w383) -> ("Objects"=w368:T4[], "3D Picture"=w369:refnum<vi>, "Position"=w361:T2)
        n156 = call <vilib>:"Create Panel.vi"("Position (0,0,0)"=w361, "error in (no error)"=w373, "Dimensions"=T2 {"X"=0.2, "Y"=0.2, "Z"=0.0}) -> ("error out"=w360:errorcluster, "Panel object"=w359:refnum<class "Panel.lvclass">)  [unwired: 7 in]
        n157 = call <vilib>:"Add Shape.vi"("error in (no error)"=w360, "Shape in"=w359) -> ("error out"=w357:errorcluster, "Shape out"=w358:refnum<class "Panel.lvclass">)  [unwired: 7 in, 1 out]
        n158 = call-dynamic "To LV 3D Pict.vi"("error in (no error)"=w357, "reference in"=w358) -> ("error out"=w372:errorcluster, "3D object ref"=w370:refnum<vi>, "reference out"=w356:refnum<class "Panel.lvclass">)  [unwired: 7 in]
        n159 = call-poly <vilib>:"Add Object.vi"("error in (no error)"=w372, "New Object In"=w370, "Scene Object In"=w369) -> ("error out"=w371:errorcluster, "New Object Out"=w365:refnum<vi>)  [unwired: 6 in, 1 out]
        n160 = Bundle By Name(cluster=T4 {"3D Pict"=refnum, "hololens"=refnum} ("new element/subarray"), "hololens"=w356, "3D Pict"=w365) -> (w364:T4)
        n161 = vi-ref "_Hololens_GaitDisplay.vi"() -> (w385:refnum<vi>)
        n162 = property class="VI"(reference=w385, error in=w371) -> (error out=w376:errorcluster, "Path"=w386:path)  [unwired: 1 out]
        n163 = Open VI Reference(type specifier VI Refnum (for type only)=refnum<vi> refnum, vi path=w386, options=128, error in (no error)=w376) -> (vi reference=w381:refnum<vi>, error out=w377:errorcluster)  [unwired: 2 in]
        n164 = call-by-ref "Start Asynchronous Call"(reference=w381, error in=w377, "Panel Shape"=w356) -> (reference out=w379:refnum<vi>, error out=w378:errorcluster)  [unwired: 11 in]
        n165 = Replace Array Subset(array=w368, new element=w364, index=4) -> (w362:T4[])
        n166 = Close Reference(reference=w379, error in (no error)=w378) -> (error out=w374:errorcluster)
        n167 = Bundle By Name(cluster=w383, "Objects"=w362) -> (w363:T6)
        n168 = property on="Panel" class="Bool"(error in=w374, "DisabledEnum"=T3."Disabled and Grayed Out" ("Disabled")) -> (error out=w387:errorcluster)  [unwired: 1 in, 1 out]
      }
      event "X rotation", "Y rotation", "Z rotation": Value Change {
        # "Applies rotation to selected object"
        n169 = event-data() -> ()  [unwired: 1 in, 1 out]
        n170 = Unbundle By Name(w396) -> ("Objects"=w398:T4[], "Tab Control"=w397:T1)
        n171 = Index Array(array=w398, index=w397) -> (element=w399:T4)
        n172 = call <vilib>:"Euler_to_Quaternion.vi"("Units (Deg)"=_Deg_Rad_typedef."Deg", "error in (no error)"=w404, "c"="X rotation", "b"="Y rotation", "a"="Z rotation") -> ("error out"=w402:errorcluster, "Quaternion"=w401:T11)  [unwired: 5 in]
        n173 = Unbundle By Name(w399) -> ("3D Pict"=w389:refnum<vi>, "hololens"=w403:refnum<class "3D_Shape.lvclass">)
        n174 = property class="3D Shapes"(reference=w403) -> (reference out=w400:refnum<class "3D_Shape.lvclass">, "properties:Shape"=w390:T12, "properties:Position"=w391:T2)  [unwired: 1 in, 1 out]
        n175 = Not A Number/Path/Refnum?(number/path/refnum=w389) -> (NaN/Path/Refnum?=w388:bool)
        n176 = case shown="False" w388 {
          tunnel: w402 -> [w430 w438]
          tunnel: w401 -> [w409 _]
          tunnel: w400 -> [w429 _]
          tunnel: w399 -> [w428 _]
          tunnel: w398 -> [w424 _]
          tunnel: w397 -> [w423 _]
          tunnel: w396 -> [w422 w437]
          tunnel: [w421 w437] -> w395
          tunnel: w389 -> [w417 _]
          tunnel: [w416 w438] -> w392
          tunnel: w391 -> [w414 _]
          tunnel: w390 -> [w413 _]
          frame False {
            # "LabVIEW cylinder must be rotated to be compatible with Hololens cylinders"
            # "Rotates 3D Picture object"
            # "Rotates Hololens object"
            # "Records the modified object"
            n177 = call <vilib>:"Move Object.vi"("Quaternion (no rotation)"=w409, "error in (no error)"=w430, "Position"=w414, "3D Object in"=w429) -> ("error out"=w418:errorcluster, "3D Object out"=w426:refnum<class "3D_Shape.lvclass">)  [unwired: 6 in]
            n178 = call <vilib>:"Clear Transformation.vi"("error in (no error)"=w418, "Object Refnum In"=w417) -> ("error out"=w412:errorcluster, "Object Refnum Out"=w410:refnum<vi>)  [unwired: 8 in]
            n179 = case shown="\"Cylinder\"" w413 {
              tunnel: w412 -> [w431 w436]
              tunnel: [w431 w435] -> w411
              tunnel: w410 -> [_ w434]
              frame "None", Default {
              }
              frame "Cylinder" {
                n180 = call <vilib>:"Rotate X-axis.vi"("Relative?"=FALSE, "error in (no error)"=w436, "angle"=90.0, "Scene Object In"=w434) -> ("error out"=w435:errorcluster)  [unwired: 6 in, 1 out]
              }
            }
            n181 = Bundle By Name(cluster=w428, "hololens"=w426) -> (w425:T4)
            n182 = call <vilib>:"quaternion_to_rotation_axis.vi"("error in"=w411, "Quaternion"=w409) -> ("error out"=w427:errorcluster, "angle (rad)"=w407:sgl, "Axis"=w408:cluster{"X":sgl, "Y":sgl, "Z":sgl})  [unwired: 7 in]
            n183 = Replace Array Subset(array=w424, new element=w425, index=w423) -> (w420:T4[])
            n184 = call <vilib>:"Rotate Object.vi"("error in (no error)"=w427, "Angle"=w407, "Axis"=w408, "Scene.Object In"=w417) -> ("error out"=w419:errorcluster, "Scene.Object Out"=w415:refnum<vi>)  [unwired: 6 in]
            n185 = Bundle By Name(cluster=w422, "Objects"=w420) -> (w421:T6)
            n186 = call <vilib>:"Set Translation.vi"("error in (no error)"=w419, "Translation"=w414, "Scene Object"=w415) -> ("error out"=w416:errorcluster)  [unwired: 7 in, 1 out]
          }
          frame True {
          }
        }
      }
      event Value Change {
        # "Records new position"
        n187 = event-data() -> ()  [unwired: 1 in, 1 out]
        n188 = Bundle By Name(cluster=w442, "Position"="Position") -> (w441:T6)
      }
    }
    n189 = Unbundle By Name(w34) -> ("Connection"=→"Hololens":bool, "3D Picture"=→"3D Picture":refnum<vi>)
    n190 = Or(x=w29, y=w31) -> (x .or. y?=w30:bool)
  }
  n191 = Unregister For Events(event registration refnum=w14, error in=w13) -> (error out=w1:errorcluster)
  n192 = call <vilib>:"Close Hololens.vi"("error in (no error)"=w1) -> ("error out"=w2:errorcluster)  [unwired: 10 in]
  n193 = call <vilib>:"Simple Error Handler.vi"("error in (no error)"=w2) -> ()  [unwired: 4 in, 5 out]
